vi "Is_MatLab_Executable_Running.vi"(3 "executable":string="EnFloSoftwareMatlabSuite") -> (0 "error out":errorcluster, 1 "Running?":bool)   [LabVIEW 2022 SP3]
panel:
  out "Standard output":string
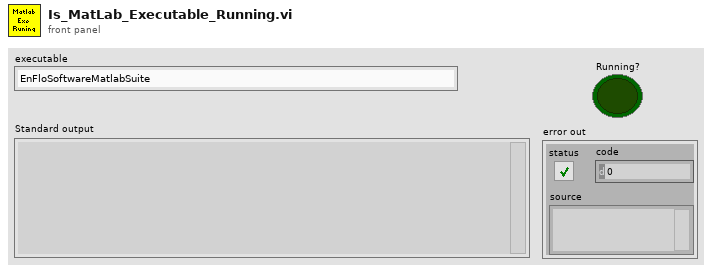
[diagram p1: front panel]
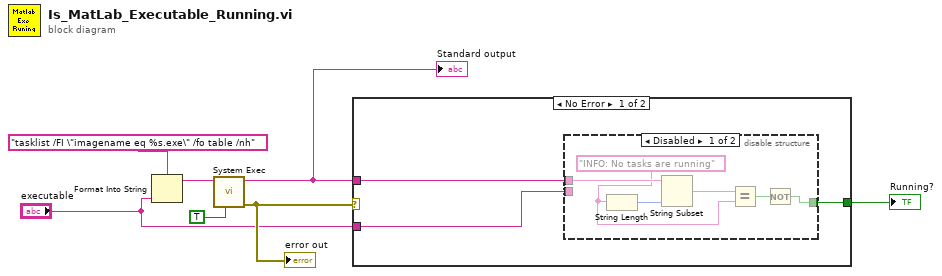
[diagram p0: block diagram]
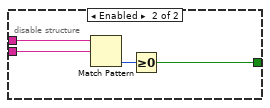
[diagram p2: hidden frame]
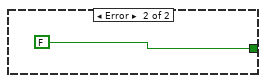
[diagram p3: hidden frame]
diagram:
  n1 = Format Into String(format string="tasklist /FI \"imagename eq %s.exe\" /fo table /nh" ("command line"), "executable") -> (resulting string=w3:string)  [unwired: 2 in, 1 out]
  n2 = call <vilib>:"System Exec.vi"("run minimized? (F)"=TRUE, "command line"=w3) -> ("error out"=w7:errorcluster, "standard output"=w6:string)  [unwired: 6 in, 2 out]
  "Standard output" <- w6
  "error out" <- w7
  n3 = case shown="No Error" w7 {
    tunnel: w6 -> [w9 _]
    tunnel: [w10 FALSE] -> w5
    tunnel: "executable" -> [w8 _]
    frame No Error {
      n4 = disable-structure shown="Disabled" {
        disable-tunnel: [w13 w18] -> w10
        disable-tunnel: w9 -> [w12 w19]
        disable-tunnel: w8 -> [_ w17]
        frame Disabled {
          w11 = "INFO: No tasks are running"
          n5 = String Length(string=w11) -> (length=w16:i32)
          n6 = String Subset(string=w12, length (rest)=w16) -> (substring=w15:string)  [unwired: 1 in]
          n7 = Equal?(x=w15, y=w11) -> (x = y?=w14:bool)
          n8 = Not(x=w14) -> (.not. x?=w13:bool)
        }
        frame Enabled {
          n9 = Match Pattern(string=w19, regular expression=w17) -> (offset past match=w20:i32)  [unwired: 1 in, 3 out]
          n10 = Greater Or Equal To 0?(x=w20) -> (x >= 0?=w18:bool)
        }
      }
    }
    frame Error {
    }
  }
  "Running?" <- w5
